vi "Write Front Panels Start State.vi"(8 "error in (no error)":errorcluster, 10 "Front Panels Start State":T1(ring)=enum."Standard", 11 "GUI View in":refnum<class "GUI View.lvclass">) -> (0 "error out":errorcluster, 3 "GUI View out":refnum<class "GUI View.lvclass">)   [LabVIEW 2023, in "GUI Views.lvlib" / "GUI View.lvclass"]
uses:
  GUI View.lvclass
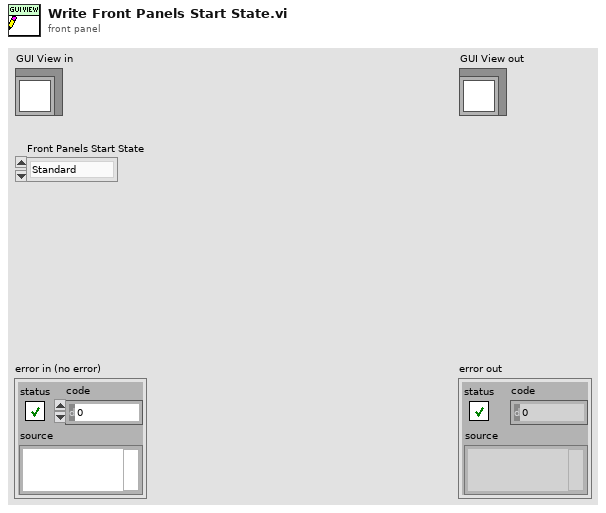
[diagram p1: front panel]
types:
  T1 = enum32{"Invalid", "Standard", "Closed", "Hidden", "Minimized", "Maximized"}
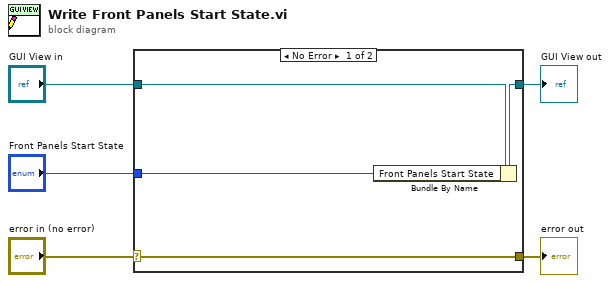
[diagram p0: block diagram]
diagram:
  n1 = case shown="No Error" "error in (no error)" {
    selector: "error in (no error)" -> [w9 w10]
    tunnel: [w9 w10] -> w4
    tunnel: [w7 w11] -> w2
    tunnel: "GUI View in" -> [w8 w11]
    tunnel: "Front Panels Start State" -> [w6 _]
    frame No Error {
      n2 = Bundle By Name(cluster=w8, "Front Panels Start State"=w6) -> (w7:refnum<class "GUI View.lvclass">)
    }
    frame Error {
    }
  }
  "error out" <- w4
  "GUI View out" <- w2
